vi "subvi Robot Read Limit Switches.vi"(2 "VISA In":refnum<visa-resource-name>) -> (0 "M1NegLim":bool, 1 "M2NegLim":bool, 3 "M1PosLim":bool, 4 "M2PosLim":bool, 5 "M3NegLim":bool, 6 "ReadOK":bool, 7 "VISA Out":refnum<visa-resource-name>, 8 "M3PosLim":bool, 9 "error out":errorcluster)   [LabVIEW 2012]
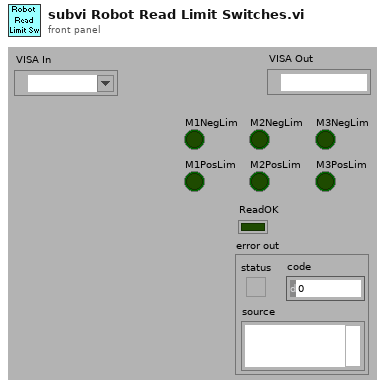
[diagram p1: front panel]
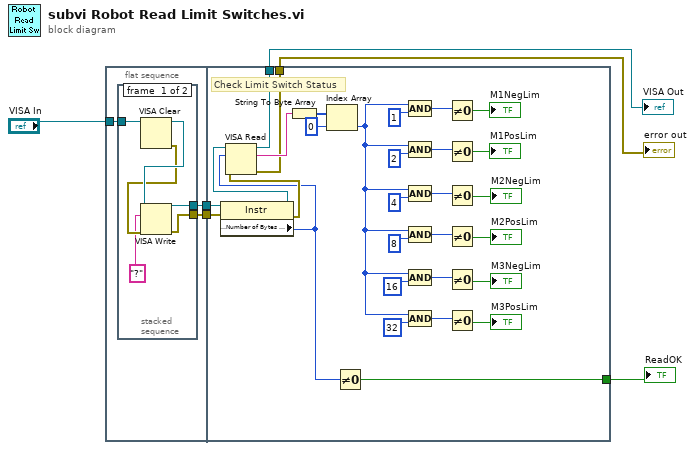
[diagram p0: block diagram]
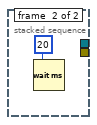
[diagram p2: hidden frame]
diagram:
  n1 = flat-sequence {
    tunnel: "VISA In" -> [w9]
    tunnel: [w8] -> w5
    tunnel: [w7] -> w4
    tunnel: w5 -> [w25]
    tunnel: w4 -> [w24]
    tunnel: [w20] -> w3
    tunnel: [w19] -> w2
    tunnel: [w17] -> w1
    frame #0 {
      n2 = stacked-sequence {
        tunnel: w9 -> [w15 _]
        tunnel: [w11 _] -> w8
        tunnel: [w10 _] -> w7
        frame #0 {
          n3 = VISA Clear(VISA resource name=w15) -> (VISA resource name out=w14:refnum<visa-resource-name>, error out=w13:errorcluster)  [unwired: 1 in]
          n4 = VISA Write(VISA resource name=w14, write buffer="?" ("Text to Send"), error in (no error)=w13) -> (VISA resource name out=w11:refnum<visa-resource-name>, error out=w10:errorcluster)  [unwired: 1 out]
        }
        frame #1 {
          n5 = Wait (ms)(milliseconds to wait=u32 20) -> ()  [unwired: 1 out]
        }
      }
    }
    frame #1 {
      # "Check Limit Switch Status"
      n6 = property class="Instr"(reference=w25, error in=w24) -> (reference out=w23:refnum<visa-resource-name>, error out=w22:errorcluster, "Serial Settings:Number of Bytes at Serial Port"=w18:u32)
      n7 = VISA Read(VISA resource name=w23, byte count=w18, error in (no error)=w22) -> (VISA resource name out=w20:refnum<visa-resource-name>, read buffer=w21:string, error out=w19:errorcluster)  [unwired: 1 out]
      n8 = String To Byte Array(string=w21) -> (unsigned byte array=w28:u8[])
      n9 = Index Array(array=w28, index=0) -> (element=w26:u8)
      n10 = Not Equal To 0?(x=w18) -> (x != 0?=w17:bool)
      n11 = Compound Arithmetic op=AND(w26, u8 1) -> (w46:u8)
      n12 = Compound Arithmetic op=AND(w26, u8 2) -> (w44:u8)
      n13 = Compound Arithmetic op=AND(w26, u8 4) -> (w42:u8)
      n14 = Compound Arithmetic op=AND(w26, u8 8) -> (w40:u8)
      n15 = Compound Arithmetic op=AND(w26, u8 16) -> (w38:u8)
      n16 = Compound Arithmetic op=AND(w26, u8 32) -> (w36:u8)
      n17 = Not Equal To 0?(x=w46) -> (x != 0?=→"M1NegLim":bool)
      n18 = Not Equal To 0?(x=w44) -> (x != 0?=→"M1PosLim":bool)
      n19 = Not Equal To 0?(x=w42) -> (x != 0?=→"M2NegLim":bool)
      n20 = Not Equal To 0?(x=w40) -> (x != 0?=→"M2PosLim":bool)
      n21 = Not Equal To 0?(x=w38) -> (x != 0?=→"M3NegLim":bool)
      n22 = Not Equal To 0?(x=w36) -> (x != 0?=→"M3PosLim":bool)
    }
  }
  "ReadOK" <- w1
  "error out" <- w2
  "VISA Out" <- w3
